vi "Generate Array Row 2016.vi"(6 "Cluster":T1, 7 "Downhole Pressure Sensor":dbl, 9 "Feet of\nStainless to be\nUsed (Count)":i32, 10 "Flow":dbl, 11 "In line Pressure Sensor":dbl format="%.2f") -> (1 "Depth Rate":dbl format="%.2f", 2 "IK":dbl, 3 "Array":dbl[](array[numeric]))   [LabVIEW 2016]
uses:
  Waterloo DAQ/controls/Kpro hydraulic measurement cluster.ctl
  KPRO_lv2015/Kpro Globals.vi
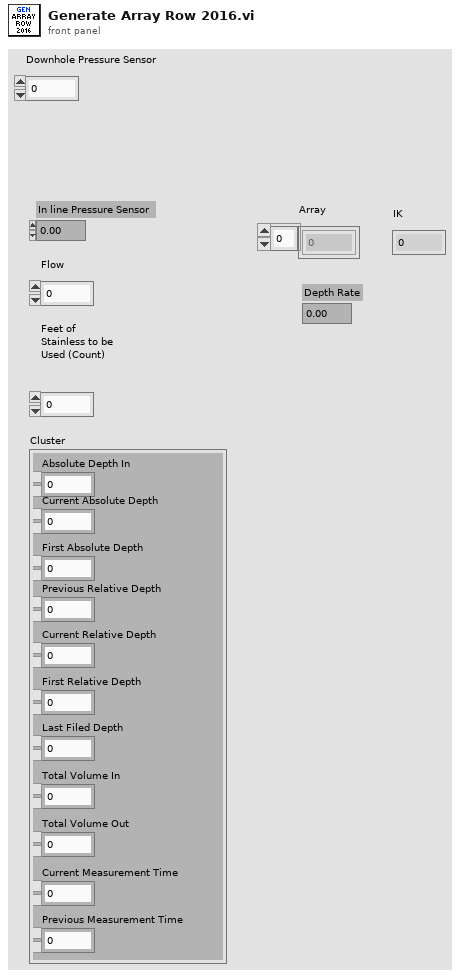
[diagram p1: front panel]
types:
  T1 = typedef "Kpro hydraulic measurement cluster.ctl" = cluster{"Absolute Depth In":dbl, "Current Absolute Depth":dbl, "First Absolute Depth":dbl, "Previous Relative Depth":dbl, "Current Relative Depth":dbl, "First Relative Depth":dbl, "Last Filed Depth":dbl, "Total Volume In":dbl, "Total Volume Out":dbl, "Current Measurement Time":dbl, "Previous Measurement Time":dbl}
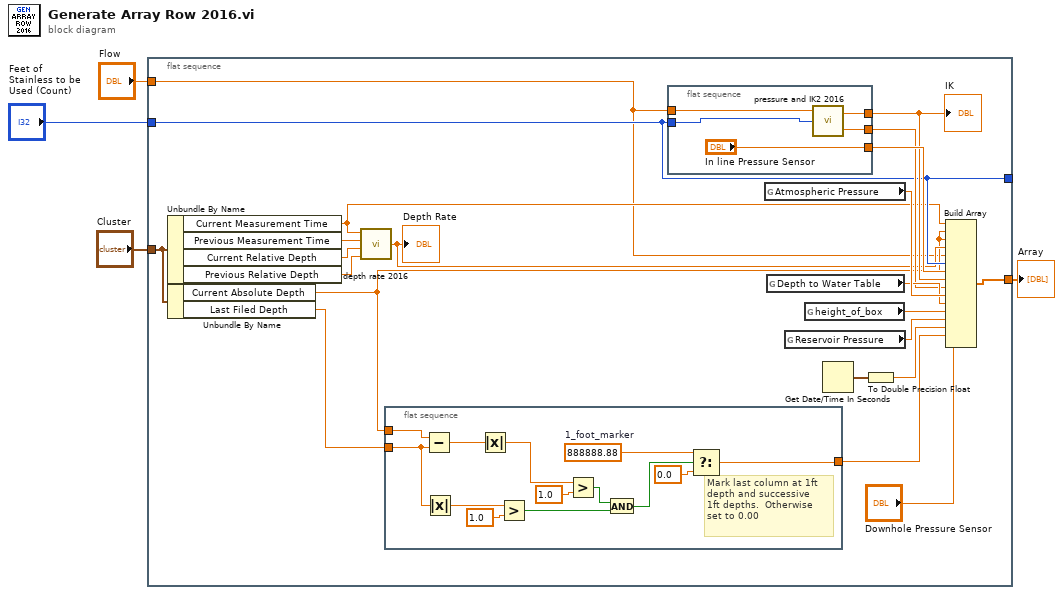
[diagram p0: block diagram]
diagram:
  n1 = flat-sequence {
    tunnel: [w26] -> w1
    tunnel: "Flow" -> [w6]
    tunnel: "Feet of\nStainless to be\nUsed (Count)" -> [w14]
    tunnel: "Cluster" -> [w10]
    tunnel: [w14] -> _
    frame #0 {
      n2 = Unbundle By Name(w10) -> ("Current Measurement Time"=w8:dbl, "Previous Measurement Time"=w11:dbl, "Current Relative Depth"=w12:dbl, "Previous Relative Depth"=w13:dbl)
      n3 = Unbundle By Name(w10) -> ("Current Absolute Depth"=w7:dbl, "Last Filed Depth"=w18:dbl)
      n4 = call "depth rate 2016.vi"("Depth Last"=w13, "Depth Current"=w12, "Time Last"=w11, "Time Current"=w8) -> ("Depth Rate"=w9:dbl)
      "Depth Rate" <- w9
      n5 = flat-sequence {
        tunnel: [w39] -> w20
        tunnel: w18 -> [w35]
        tunnel: w7 -> [w32]
        frame #0 {
          w41 = 888888.88  # 1_foot_marker
          # "Mark last column at 1ft \ndepth and successive\n1ft depths.  Otherwise\nset to 0.00"
          n6 = Subtract(x=w32, y=w35) -> (x-y=w44:dbl)
          n7 = Absolute Value(x=w35) -> (abs(x)=w33:dbl)
          n8 = Absolute Value(x=w44) -> (abs(x)=w42:dbl)
          n9 = Greater?(x=w33, y=1.0) -> (0:w36:bool)
          n10 = Greater?(x=w42, y=1.0) -> (0:w37:bool)
          n11 = And(x=w37, y=w36) -> (x .and. y?=w38:bool)
          n12 = Select(t=w41, s=w38, f=0.0) -> (s? t:f=w39:dbl)
        }
      }
      n13 = flat-sequence {
        tunnel: [w31] -> w15
        tunnel: ["In line Pressure Sensor"] -> w17
        tunnel: w6 -> [w30]
        tunnel: [w29] -> w16
        tunnel: w14 -> [w28]
        frame #0 {
          n14 = call "pressure and IK2 2016.vi"("Ft. of SS"=w28, "flow"=w30) -> ("Corrected Headloss"=w31:dbl, "IK"=w29:dbl)  [unwired: 1 in]
        }
      }
      n15 = global read "Kpro Globals.vi" "Atmospheric Pressure"() -> (w25:dbl)
      n16 = global read "Kpro Globals.vi" "Depth to Water Table"() -> (w23:dbl)
      n17 = global read "Kpro Globals.vi" "Reservoir Pressure"() -> (w24:dbl)
      n18 = global read "Kpro Globals.vi" "height_of_box"() -> (w22:dbl)
      n19 = Get Date/Time In Seconds() -> (seconds since 1Jan1904=w19:timestamp)
      n20 = To Double Precision Float(number=w19) -> (double precision float=w21:dbl)
      n21 = Build Array(w8, w7, w7, w9, w6, w14, w17, w16, w15, w25, w23, w22, w24, w21, w20, "Downhole Pressure Sensor") -> (w26:dbl[])
      "IK" <- w16
    }
  }
  "Array" <- w1
